vi "Write listener ID.vi"(8 "error in (no error)":errorcluster, 10 "listener ID":refnum<k5>, 11 "RemoteControl.STM in":refnum<class "RemoteControl.STM.lvclass">) -> (0 "error out":errorcluster, 3 "RemoteControl.STM out":refnum<class "RemoteControl.STM.lvclass">)   [LabVIEW 2020, in "RemoteControl.STM.lvclass"]
uses:
  RemoteControl.STM.lvclass
  RemoteControl.STM.lvclass/RemoteControl.STM.ctl
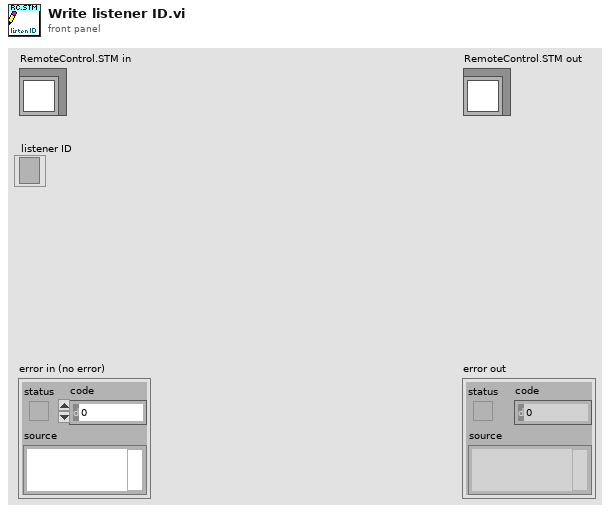
[diagram p1: front panel]
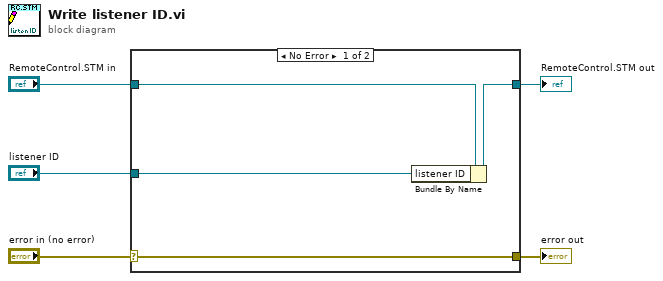
[diagram p0: block diagram]
diagram:
  n1 = case shown="No Error" "error in (no error)" {
    selector: "error in (no error)" -> [w9 w10]
    tunnel: [w9 w10] -> w4
    tunnel: [w7 w11] -> w2
    tunnel: "RemoteControl.STM in" -> [w8 w11]
    tunnel: "listener ID" -> [w6 _]
    frame No Error {
      n2 = Bundle By Name(cluster=w8, "listener ID"=w6) -> (w7:refnum<class "RemoteControl.STM.lvclass">)
    }
    frame Error {
    }
  }
  "error out" <- w4
  "RemoteControl.STM out" <- w2
